vi "Read Exception Status.vi"(8 "error in (no error)":errorcluster, 11 "Modbus master in":refnum<class "Modbus Master.lvclass">) -> (0 "error out":errorcluster, 2 "exception status":u8, 3 "Modbus master out":refnum<class "Modbus Master.lvclass">)   [LabVIEW 2015, in "Modbus Master.lvclass"]
doc: "Reads the exception status of a Modbus slave. The exception status is a set of eight status bits. Each status bit represents an exception."
uses:
  <vilib>/Modbus/master/Modbus Master.lvclass
  <vilib>/Modbus/subvis/Modbus API/Modbus API.lvclass/Modbus API.ctl
  <vilib>/Modbus/subvis/Transmission Data Unit (ADU)/Serial Data Unit/Serial Data Unit.lvclass
  <vilib>/Modbus/master/Modbus Master.lvclass/Modbus Master.ctl
  <vilib>/Modbus/subvis/Protocol/Interfaces/Network Master/Network Master.lvclass
  <vilib>/Modbus/subvis/Transmission Data Unit (ADU)/Transmission Data Unit/Transmission Data Unit.lvclass
  <vilib>/Modbus/subvis/Modbus API/Modbus API.lvclass
  <vilib>/Modbus/subvis/Data and Functions/Master Function Definition/Master Function Definition.lvlib
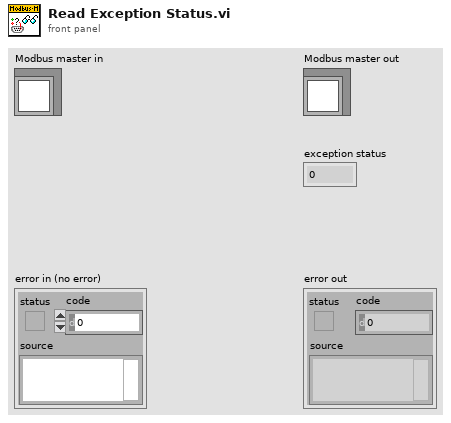
[diagram p1: front panel]
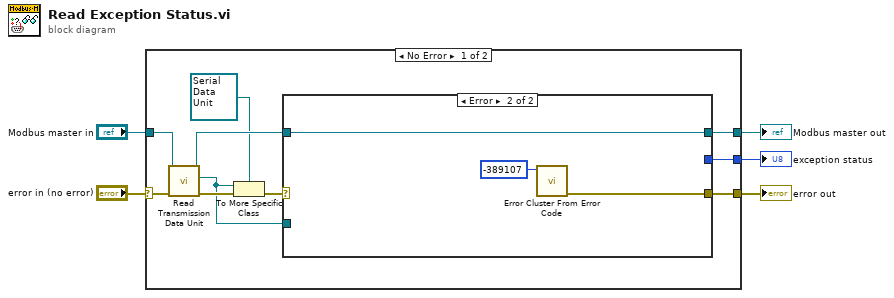
[diagram p0: block diagram]
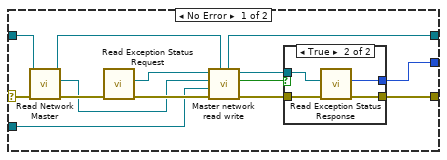
[diagram p2: hidden frame]
diagram:
  n1 = case shown="No Error" "error in (no error)" {
    selector: "error in (no error)" -> [w10 w38]
    tunnel: [w14 w39] -> w5
    tunnel: "Modbus master in" -> [w13 w39]
    tunnel: [w12 _] -> w3
    tunnel: [w11 w38] -> w2
    frame No Error {
      n2 = call <vilib>:"Read Transmission Data Unit.vi"("error in (no error)"=w10, "Modbus instance in"=w13) -> ("error out"=w9:errorcluster, "transmission data unit"=w8:refnum<class "Transmission Data Unit.lvclass">, "Modbus instance out"=w15:refnum<class "Modbus Master.lvclass">)  [unwired: 7 in]
      n3 = To More Specific Class(target class=refnum<class "Serial Data Unit.lvclass"> refnum ("Serial Data Unit"), reference=w8, error in=w9) -> (error out=w6:errorcluster)  [unwired: 1 out]
      n4 = case shown="Error" w6 {
        selector: w6 -> [w16 _]
        tunnel: w15 -> [w29 w36]
        tunnel: [w24 w36] -> w14
        tunnel: [w22 _] -> w12
        tunnel: [w19 w37] -> w11
        tunnel: w8 -> [w17 _]
        frame No Error {
          n5 = call <vilib>:"Read Network Master.vi"("error in (no error)"=w16, "Modbus master in"=w29) -> ("error out"=w26:errorcluster, "network master"=w23:refnum<class "Network Master.lvclass">, "Modbus master out"=w25:refnum<class "Modbus Master.lvclass">)  [unwired: 7 in]
          n6 = call <vilib>:"Read Exception Status Request.vi"("error in (no error)"=w26) -> ("error out"=w28:errorcluster, "Modbus data unit out"=w27:refnum<class "Modbus Data Unit (PDU).lvclass">)  [unwired: 9 in]
          n7 = call <vilib>:"Master network read write.vi"("Modbus master in"=w25, "error in (no error)"=w28, "transmission data unit in"=w17, "network master in"=w23, "Modbus data unit in"=w27) -> ("error out"=w20:errorcluster, "PDU valid?"=w18:bool, "Modbus data unit out"=w21:refnum<class "Modbus Data Unit (PDU).lvclass">, "Modbus master out"=w24:refnum<class "Modbus Master.lvclass">)  [unwired: 3 in]
          n8 = case shown="True" w18 {
            tunnel: [_ w34] -> w22
            tunnel: w21 -> [_ w33]
            tunnel: w20 -> [w30 w32]
            tunnel: [w30 w31] -> w19
            frame False {
            }
            frame True {
              n9 = call <vilib>:"Read Exception Status Response.vi"("error in (no error)"=w32, "Modbus data unit in"=w33) -> ("error out"=w31:errorcluster, "exception status"=w34:u8)  [unwired: 8 in]
            }
          }
        }
        frame Error {
          n10 = call <vilib>:"Error Cluster From Error Code.vi"("error code (0)"=-389107) -> ("error out"=w37:errorcluster)  [unwired: 8 in]
        }
      }
    }
    frame Error {
    }
  }
  "error out" <- w2
  "Modbus master out" <- w5
  "exception status" <- w3
